vi "ETH 12 Main.vi"(7 "ETH12 Q":refnum<queue>, 8 "error in":errorcluster, 11 "data in":string) -> (0 "error out":errorcluster)   [LabVIEW 2022 SP3]
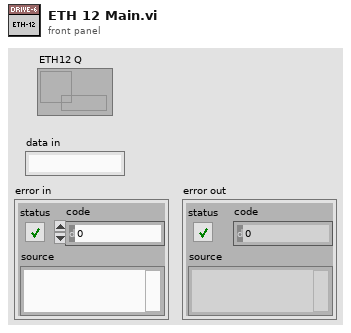
[diagram p1: front panel]
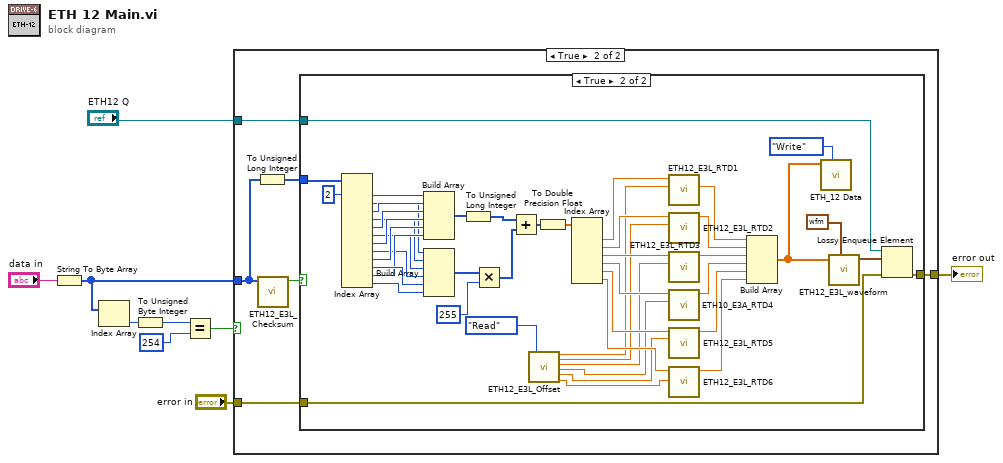
[diagram p0: block diagram]
diagram:
  n1 = String To Byte Array(string="data in") -> (unsigned byte array=w4:u8[])
  n2 = Index Array(array=w4) -> (element=w9:u8)  [unwired: 1 in]
  n3 = To Unsigned Byte Integer(number=w9) -> (unsigned 8bit integer=w8:u8)
  n4 = Equal?(x=w8, y=u8 254) -> (x = y?=w5:bool)
  n5 = case shown="True" w5 {
    tunnel: w4 -> [_ w15]
    tunnel: "ETH12 Q" -> [_ w13]
    tunnel: "error in" -> [w10 w12]
    tunnel: [w10 w11] -> w1
    frame False {
    }
    frame True {
      n6 = To Unsigned Long Integer(number=w15) -> (unsigned 32bit integer=w14:u32[])
      n7 = call "ETH12_E3L_Checksum.vi"("unsigned byte array"=w15) -> ("Checksum"=w16:bool)  [unwired: 10 in]
      n8 = case shown="True" w16 {
        tunnel: w14 -> [_ w20]
        tunnel: w13 -> [_ w44]
        tunnel: w12 -> [w17 w42]
        tunnel: [w17 w41] -> w11
        frame False {
        }
        frame True {
          n9 = Index Array(array=w20, index #1=2 ("index")) -> (element #1=w24:u32, element #2=w25:u32, element #3=w26:u32, element #4=w27:u32, element #5=w28:u32, element #6=w29:u32, element #7=w30:u32, element #8=w31:u32, element #9=w32:u32, element #10=w35:u32, element #11=w33:u32, element #12=w34:u32)  [unwired: 11 in]
          n10 = Build Array(w24, w26, w28, w30, w32, w33) -> (w23:u32[])
          n11 = Build Array(w25, w27, w29, w31, w35, w34) -> (w22:u32[])
          n12 = To Unsigned Long Integer(number=w23) -> (unsigned 32bit integer=w37:u32[])
          n13 = Multiply(x=w22, y=u32 255) -> (x*y=w38:u32[])
          n14 = Add(x=w37, y=w38) -> (x+y=w36:u32[])
          n15 = call "ETH12_E3L_Offset.vi"("Write/Read"=enum16{"Write", "Read"}."Read") -> ("RTD1 Offset Out"=w57:dbl, "RTD2 Offset Out"=w56:dbl, "RTD3 Offset Out"=w55:dbl, "RTD4 Offset out"=w54:dbl, "RTD5 Offset out"=w53:dbl, "RTD6 Offset  out"=w52:dbl)  [unwired: 13 in]
          n16 = To Double Precision Float(number=w36) -> (double precision float=w19:dbl[])
          n17 = Index Array(array=w19) -> (element #1=w64:dbl, element #2=w63:dbl, element #3=w62:dbl, element #4=w61:dbl, element #5=w60:dbl, element #6=w59:dbl)  [unwired: 6 in]
          n18 = call "ETH12_E3L_RTD1.vi"("RTD 1 Off"=w57, "Input Variable"=w64) -> ("RTD Value"=w51:dbl)  [unwired: 9 in]
          n19 = call "ETH12_E3L_RTD2.vi"("RTD 2 Off"=w56, "Input Variable"=w63) -> ("RTD Value"=w50:dbl)  [unwired: 9 in]
          n20 = call "ETH12_E3L_RTD3.vi"("RTD 3 Off"=w55, "Input Variable"=w62) -> ("RTD Value"=w49:dbl)  [unwired: 9 in]
          n21 = call "ETH10_E3A_RTD4.vi"("RTD 4 Off"=w54, "Input Variable"=w61) -> ("RTD Value"=w48:dbl)  [unwired: 9 in]
          n22 = call "ETH12_E3L_RTD5.vi"("RTD 5 Off"=w53, "Input Variable"=w60) -> ("RTD Value"=w47:dbl)  [unwired: 9 in]
          n23 = call "ETH12_E3L_RTD6.vi"("RTD 6 Off"=w52, "Input Variable"=w59) -> ("RTD Value"=w46:dbl)  [unwired: 9 in]
          n24 = Build Array(w51, w50, w49, w48, w47, w46) -> (w39:dbl[])
          n25 = call "ETH_12 Data.vi"("Enum"=enum16{"Read", "Write"}."Write", "ETH_12"=w39) -> ()  [unwired: 8 in, 2 out]
          n26 = call "ETH12_E3L_waveform.vi"("Waveform"=waveform(dbl) {"t0"=timestamp(0 s since 1904-01-01), "dt"=0.001, "Y"=[]}, "Array in"=w39) -> ("Array out"=w43:waveform(dbl)[])  [unwired: 9 in]
          n27 = Lossy Enqueue Element(queue=w44, element=w43, error in (no error)=w42) -> (error out=w41:errorcluster)  [unwired: 3 out]
        }
      }
    }
  }
  "error out" <- w1
